vi "Double Fulfill Error.vi"(8 "error in (no error)":errorcluster) -> (0 "error out":errorcluster)   [LabVIEW 2017, in "Unit Tests.lvlib"]
uses:
  Unit Tests.lvlib
  <vilib>/addons/_JKI Toolkits/Caraya/classes/Test/Test.lvclass
  <vilib>/addons/_JKI Toolkits/Caraya/classes/Assert/Assert.lvclass
  Promise/Promise/Promise.lvclass
  35a20ce0-7d2e-463e-9af8-0ba737e69b1d.vi
  a7f08ccb-5f26-4e0b-90f0-4ca9355b146f.vi
  813482e7-0724-4208-95d9-3408344fa375.vi
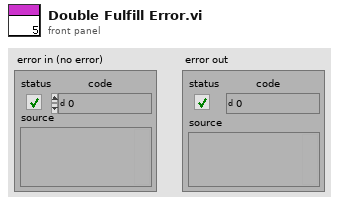
[diagram p1: front panel]
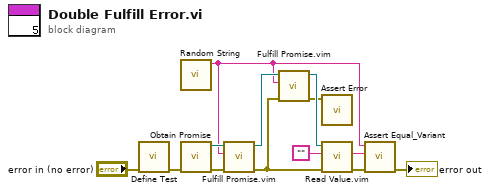
[diagram p0: block diagram]
diagram:
  n1 = call <vilib>:"Define Test.vi"("error in (no error)"="error in (no error)") -> ("error out"=w10:errorcluster)  [unwired: 10 in]
  n2 = call "Random String.vi"() -> ("string"=w7:string)  [unwired: 11 in]
  n3 = call "Obtain Promise.vi"("error in (no error)"=w10) -> ("error out"=w11:errorcluster, "Promise out"=w9:refnum<class "Promise.lvclass">)  [unwired: 8 in, 1 out]
  n4 = call "Fulfill Promise.vim"("error in (no error)"=w11, "Value"=w7, "Promise in"=w9) -> ("error out"=w1:errorcluster, "Promise out"=w8:refnum<class "Promise.lvclass">)  [unwired: 7 in]
  n5 = call "Fulfill Promise.vim"("error in (no error)"=w1, "Value"=w7, "Promise in"=w8) -> ("error out"=w2:errorcluster, "Promise out"=w5:refnum<class "Promise.lvclass">)  [unwired: 7 in]
  n6 = call <vilib>:"Assert Error.vi"("Error?"=w2) -> ()  [unwired: 10 in, 1 out]
  n7 = call "Read Value.vim"("error in (no error)"=w1, "Default Value"="", "Future in"=w5) -> ("error out"=w4:errorcluster, "Value"=w3:string)  [unwired: 5 in, 2 out]
  n8 = call <vilib>:"Assert Equal_Variant.vi"("error in (no error)"=w4, "Y"=w3, "X"=w7) -> ("error out"=→"error out":errorcluster)  [unwired: 8 in]
